vi "Test Load Virtual NEO480 cRIO XNET.vi"(11 "Test Case In":refnum<class "Test Instrument Manager.lvclass">) -> (0 "error out":errorcluster, 3 "Test Case Out":refnum<class "Test Instrument Manager.lvclass">)   [LabVIEW 2024, in "Test Instrument Manager.lvclass"]
uses:
  Test Instrument Manager.lvclass
  Test Instrument Manager.lvclass/Test Instrument Manager.ctl
  <vilib>/Astemes/LUnit/Test Case.lvclass
  Source/Instrument Manager/Instrument Manager.lvclass
  Source/Interfaces/IRead Temperature/IRead Temperature.lvclass
  Source/Interfaces/IVirtual Instrument/IVirtual Instrument.lvclass
  Source/Interfaces/IReadPressure/IRead Pressure.lvclass
  Source/Interfaces/IRead Dew Point/IRead Dew Point.lvclass
  Source/Interfaces/IRead Humidity/IRead Humidity.lvclass
  Source/Interfaces/IRead H2O Concentration/IRead H2O Concentration.lvclass
  Source/Interfaces/IRunnable/IRunnable.lvclass
panel:
  out "Time Stamp c":timestamp format="%<%x %.3X>T"
  out "H2O Concentration":dbl format="%d Vol.-%"
  out "Absolute Humidity":dbl format="%.1f g/m³"
  out "Time Stamp h":timestamp format="%<%x %.3X>T"
  out "iteration":i32
  out "Dew Point":dbl format="%.2f °C"
  out "Time Stamp d":timestamp format="%<%x %.3X>T"
  out "Time Stamp p":timestamp format="%<%x %.3X>T"
  out "Pressure":dbl format="%d mbar a"
  out "Temperature":dbl format="%.2f °C"
  out "Time Stamp t":timestamp format="%<%x %.3X>T"
  in  "stop":bool
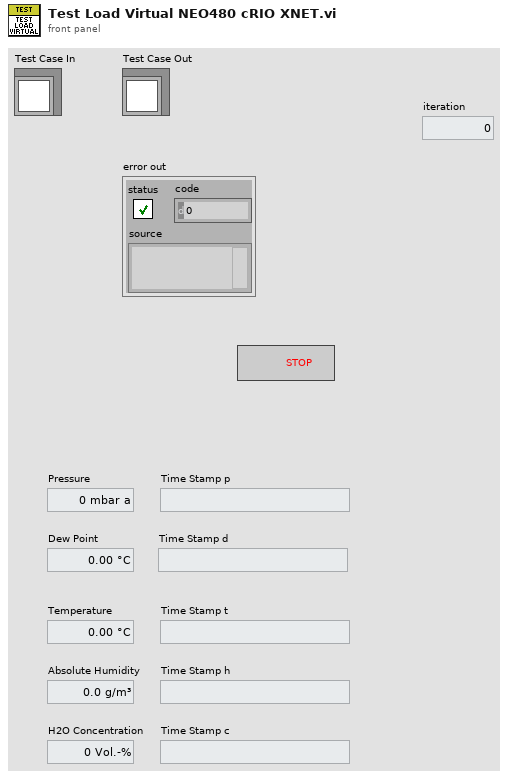
[diagram p1: front panel]
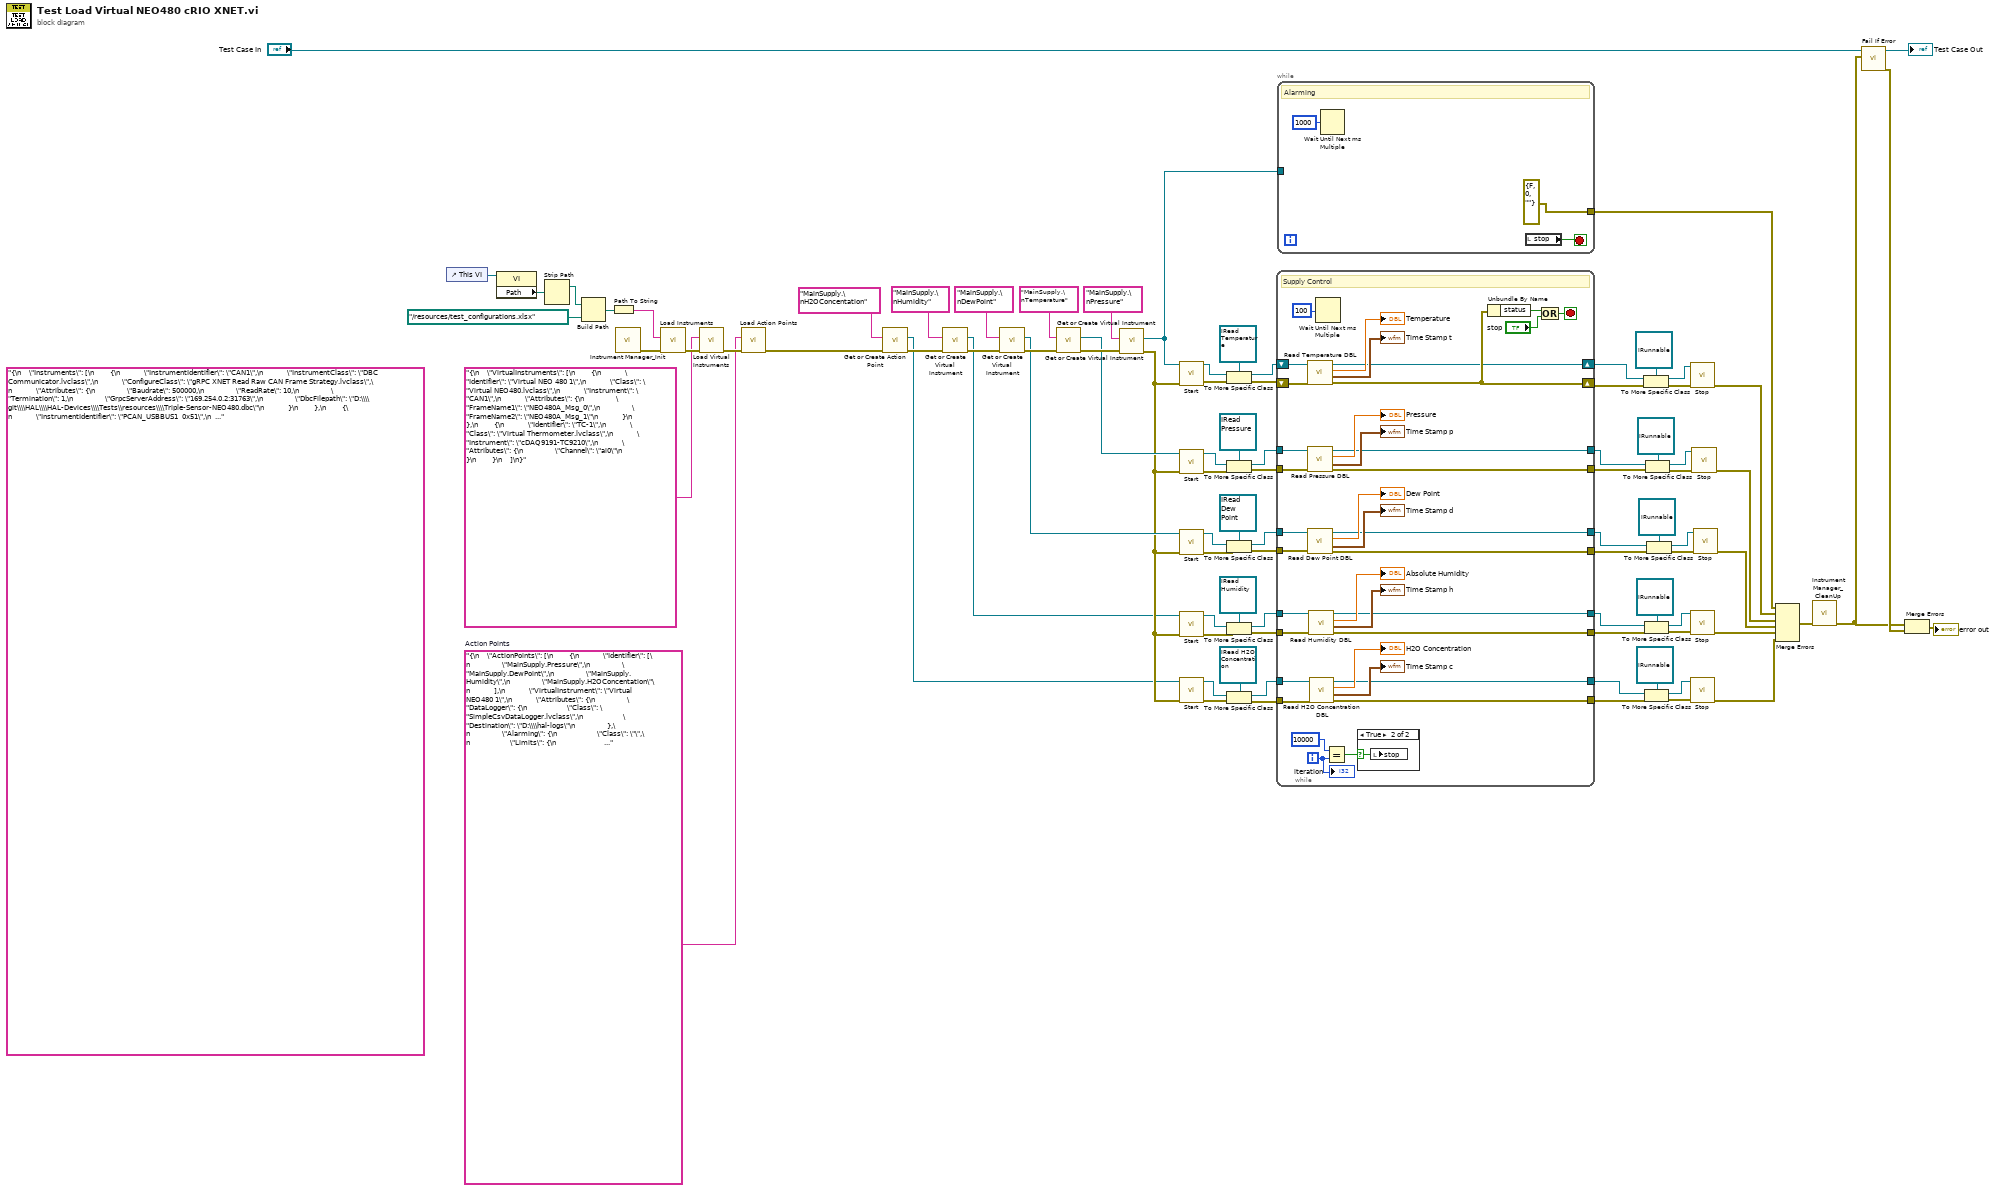
[diagram p0: block diagram]
diagram:
  w1 = "{\n    \"ActionPoints\": [\n        {\n            \"Identifier\": [\n                \"MainSupply.Pressure\",\n                \"MainSupply.DewPoint\",\n                \"MainSupply.Humidity\",\n                \"MainSupply.H2OConcentation\"\n            ],\n            \"VirtualInstrument\": \"Virtual NEO480 1\",\n            \"Attributes\": {\n                \"DataLogger\": {\n                    \"Class\": \"SimpleCsvDataLogger.lvclass\",\n                    \"Destination\": \"D:\\\\hal-logs\"\n                },\n                \"Alarming\": {\n                    \"Class\": \"\",\n                    \"Limits\": {\n                        \"Upper\": 999,\n                        \"Lower\": 0\n                    }\n                }\n            }\n        },\n        {\n            \"Identifier\": [\n                \"MainSupply.Temperature\"\n            ],\n            \"VirtualInstrument\": \"Virtual NEO480 1\",\n            \"Attributes\": {\n                \"DataLogger\": {\n                    \"Class\": \"SimpleCsvDataLogger.lvclass\",\n                    \"Destination\": \"D:\\\\hal-logs\"\n                },\n                \"Alarming\": {\n                    \"Class\": \"\",\n                    \"Limits\": {\n                        \"Upper\": 32,\n                        \"Lower\": 0\n                    }\n                }\n            }\n        }\n    ]\n}"  # Action Points
  (unwired) "{\n    \"Instruments\": [\n        {\n            \"InstrumentIdentifier\": \"CAN1\",\n            \"InstrumentClass\": \"DBC Communicator.lvclass\",\n            \"ConfigureClass\": \"gRPC XNET Read Raw CAN Frame Strategy.lvclass\",\n            \"Attributes\": {\n                \"Baudrate\": 500000,\n                \"ReadRate\": 10,\n                \"Termination\": 1,\n                \"GrpcServerAddress\": \"169.254.0.2:31763\",\n                \"DbcFilepath\": \"D:\\\\git\\\\HAL\\\\HAL-Devices\\\\Tests\\resources\\\\Triple-Sensor-NEO480.dbc\"\n            }\n        },\n        {\n            \"InstrumentIdentifier\": \"PCAN_USBBUS1  0x51\",\n            \"InstrumentClass\": \"DBC Communicator.lvclass\",\n            \"ConfigureClass\": \"PCAN Read Raw CAN Frame Strategy.lvclass\",\n            \"Attributes\": {\n                \"Baudrate\": 500000,\n                \"ReadRate\": 10,\n                \"DbcFilepath\": \"D:\\\\git\\\\HAL\\\\HAL-Devices\\\\Tests\\resources\\\\Triple-Sensor-NEO480.dbc\"\n            }\n        },\n        {\n            \"InstrumentIdentifier\": \"cDAQ9191-TC9210\",\n            \"InstrumentClass\": \"Thermometer Multichannel.lvclass\",\n            \"ConfigureClass\": \"DAQmx Thermocouple Continuous Read Strategy.lvclass\",\n            \"Attributes\": {\n                \"ReadRate\": 10,\n                \"Channels\": [\n                    {\n                        \"Name\": \"ai0\",\n                        \"Enabled\": true,\n                        \"Minimum Value\": 0,\n                        \"Maximum Value\": 100,\n                        \"Thermocouple Type\": \"J\",\n                        \"Units\": \"Deg C\",\n                        \"CJC Channel\": \"\",\n                        \"CJC Source\": \"Constant Value\",\n                        \"CJC Value\": 25\n                    }\n                ],\n                \"Timing\": {\n                    \"Type\": \"Sample Clock\",\n                    \"Samples per Channel\": 1000,\n                    \"Sample Mode\": \"Continuous Samples\",\n                    \"Sample Rate\": 10,\n                    \"Sample Clock Source\": \"OnboardClock\",\n                    \"Active Edge\": \"Rising\"\n                },\n                \"Trigger\": {\n                    \"Trigger Type\": \"No Trigger\"\n                }\n            }\n        }\n    ]\n}" ("Source")
  n1 = control-ref of="This VI"() -> (w38:refnum<vi>)
  n2 = property class="VI"(reference=w38) -> ("Path"=w37:path)  [unwired: 1 in, 2 out]
  n3 = Strip Path(path=w37) -> (stripped path=w36:path)  [unwired: 1 out]
  n4 = Build Path(base path=w36, name or relative path=path "../resources/test_configurations.xlsx") -> (appended path=w34:path)
  n5 = Path To String(path=w34) -> (string=w33:string)
  n6 = call "Instrument Manager_Init.vi"() -> ("Error Out"=w84:errorcluster)  [unwired: 10 in, 1 out]
  n7 = call "Load Instruments.vi"("Error In"=w84, "Source"=w33) -> ("Error Out"=w81:errorcluster)  [unwired: 9 in]
  n8 = call "Load Virtual Instruments.vi"("Error In"=w81, "Source"="{\n    \"VirtualInstruments\": [\n        {\n            \"Identifier\": \"Virtual NEO 480 1\",\n            \"Class\": \"Virtual NEO480.lvclass\",\n            \"Instrument\": \"CAN1\",\n            \"Attributes\": {\n                \"FrameName1\": \"NEO480A_Msg_0\",\n                \"FrameName2\": \"NEO480A_Msg_1\"\n            }\n        },\n        {\n            \"Identifier\": \"TC-1\",\n            \"Class\": \"Virtual Thermometer.lvclass\",\n            \"Instrument\": \"cDAQ9191-TC9210\",\n            \"Attributes\": {\n                \"Channel\": \"ai0\"\n            }\n        }\n    ]\n}") -> ("Error Out"=w53:errorcluster)  [unwired: 9 in]
  n9 = call "Load Action Points.vi"("Error In"=w53, "Source"=w1) -> ("Error Out"=w2:errorcluster)  [unwired: 9 in]
  n10 = call "Get or Create Action Point.vi"("Error In"=w2, "Action Point Identifier"="MainSupply.\nH2OConcentation" ("Virtual Instrument Identifier")) -> ("Error Out"=w6:errorcluster, "IAction Point"=w3:refnum<class "IVirtual Instrument.lvclass">)  [unwired: 8 in]
  n11 = call "Get or Create Virtual Instrument.vi"("Error In"=w6, "Virtual Instrument Identifier"="MainSupply.\nHumidity") -> ("Error Out"=w16:errorcluster, "IVritual Instrument"=w4:refnum<class "IVirtual Instrument.lvclass">)  [unwired: 8 in]
  n12 = call "Get or Create Virtual Instrument.vi"("Error In"=w16, "Virtual Instrument Identifier"="MainSupply.\nDewPoint" ("Instrument Identifier")) -> ("Error Out"=w52:errorcluster, "IVritual Instrument"=w48:refnum<class "IVirtual Instrument.lvclass">)  [unwired: 8 in]
  n13 = call "Get or Create Virtual Instrument.vi"("Error In"=w52, "Virtual Instrument Identifier"="MainSupply.\nTemperature") -> ("Error Out"=w79:errorcluster, "IVritual Instrument"=w54:refnum<class "IVirtual Instrument.lvclass">)  [unwired: 8 in]
  n14 = call "Get or Create Virtual Instrument.vi"("Error In"=w79, "Virtual Instrument Identifier"="MainSupply.\nPressure" ("Instrument Identifier")) -> ("Error Out"=w18:errorcluster, "IVritual Instrument"=w39:refnum<class "IVirtual Instrument.lvclass">)  [unwired: 8 in]
  n15 = call-dynamic "Start.vi"("error in"=w18, "IRunnable in"=w39) -> ("error out"=w72:errorcluster, "IRunnable out"=w73:refnum<class "IVirtual Instrument.lvclass">)  [unwired: 8 in]
  n16 = call-dynamic "Start.vi"("error in"=w18, "IRunnable in"=w54) -> ("error out"=w69:errorcluster, "IRunnable out"=w68:refnum<class "IVirtual Instrument.lvclass">)  [unwired: 8 in]
  n17 = call-dynamic "Start.vi"("error in"=w18, "IRunnable in"=w48) -> ("error out"=w59:errorcluster, "IRunnable out"=w60:refnum<class "IVirtual Instrument.lvclass">)  [unwired: 8 in]
  n18 = call-dynamic "Start.vi"("error in"=w18, "IRunnable in"=w4) -> ("error out"=w31:errorcluster, "IRunnable out"=w30:refnum<class "IVirtual Instrument.lvclass">)  [unwired: 8 in]
  n19 = call-dynamic "Start.vi"("error in"=w18, "IRunnable in"=w3) -> ("error out"=w19:errorcluster, "IRunnable out"=w17:refnum<class "IVirtual Instrument.lvclass">)  [unwired: 8 in]
  n20 = To More Specific Class(target class=refnum<class "IRead Temperature.lvclass"> refnum ("IRead Temperature.lvclass"), reference=w73, error in=w72) -> (specific class reference=w70:refnum<class "IRead Temperature.lvclass">, error out=w71:errorcluster)
  n21 = To More Specific Class(target class=refnum<class "IRead Pressure.lvclass"> refnum ("IRead Pressure.lvclass"), reference=w68, error in=w69) -> (specific class reference=w56:refnum<class "IRead Pressure.lvclass">, error out=w55:errorcluster)
  n22 = To More Specific Class(target class=refnum<class "IRead Dew Point.lvclass"> refnum ("IRead Dew Point.lvclass"), reference=w60, error in=w59) -> (specific class reference=w57:refnum<class "IRead Dew Point.lvclass">, error out=w58:errorcluster)
  n23 = To More Specific Class(target class=refnum<class "IRead Humidity.lvclass"> refnum ("IRead Humidity.lvclass"), reference=w30, error in=w31) -> (specific class reference=w27:refnum<class "IRead Humidity.lvclass">, error out=w28:errorcluster)
  n24 = To More Specific Class(target class=refnum<class "IRead H2O Concentration.lvclass"> refnum ("IRead H2O Concentration.lvclass"), reference=w17, error in=w19) -> (specific class reference=w15:refnum<class "IRead H2O Concentration.lvclass">, error out=w20:errorcluster)
  n25 = while {
    shift-right: [w118] -> w77
    shift-left: w70 -> [w116]
    shift-right: [w119] -> w86
    shift-left: w71 -> [w117]
    tunnel: w58 -> [w110]
    tunnel: w57 -> [w109]
    tunnel: w56 -> [w108]
    tunnel: w55 -> [w107]
    tunnel: [w106] -> w41
    tunnel: [w105] -> w42
    tunnel: [w104] -> w43
    tunnel: [w103] -> w44
    tunnel: w28 -> [w101]
    tunnel: w27 -> [w100]
    tunnel: [w99] -> w26
    tunnel: [w96] -> w25
    tunnel: w20 -> [w95]
    tunnel: [w92] -> w10
    tunnel: w15 -> [w91]
    tunnel: [w90] -> w9
    i -> [w102]
    stop <- w123 stop-if-true
    # "Supply Control"
    n26 = call-dynamic "Read Temperature DBL.vi"("error in"=w117, "IRead Temperature in"=w116) -> ("error out"=w119:errorcluster, "Time Stamp"=→"Time Stamp t":timestamp, "Temperature"=→"Temperature":dbl, "IRead Temperature out"=w118:refnum<class "IRead Temperature.lvclass">)  [unwired: 6 in]
    n27 = call-dynamic "Read Pressure DBL.vi"("error in"=w107, "IRead Pressure in"=w108) -> ("error out"=w106:errorcluster, "Time Stamp"=→"Time Stamp p":timestamp, "Pressure"=→"Pressure":dbl, "IRead Pressure out"=w105:refnum<class "IRead Pressure.lvclass">)  [unwired: 6 in]
    n28 = call-dynamic "Read Dew Point DBL.vi"("error in"=w110, "IRead Dew Point in"=w109) -> ("error out"=w103:errorcluster, "Time Stamp"=→"Time Stamp d":timestamp, "Dew Point"=→"Dew Point":dbl, "IRead Dew Point out"=w104:refnum<class "IRead Dew Point.lvclass">)  [unwired: 6 in]
    n29 = call-dynamic "Read Humidity DBL.vi"("error in"=w101, "IRead Absolute Humidity in"=w100) -> ("error out"=w99:errorcluster, "Time Stamp"=→"Time Stamp h":timestamp, "Humidity"=→"Absolute Humidity":dbl, "IRead Absolute Humidity out"=w96:refnum<class "IRead Humidity.lvclass">)  [unwired: 6 in]
    n30 = call-dynamic "Read H2O Concentration DBL.vi"("error in"=w95, "IRead Water Concentration in"=w91) -> ("error out"=w92:errorcluster, "Time Stamp"=→"Time Stamp c":timestamp, "H2O Concentration"=→"H2O Concentration":dbl, "IRead Water Concentration out"=w90:refnum<class "IRead H2O Concentration.lvclass">)  [unwired: 6 in]
    n31 = Wait Until Next ms Multiple(millisecond multiple=u32 100) -> ()  [unwired: 1 out]
    n32 = Equal?(x=10000, y=w102) -> (x = y?=w115:bool)
    n33 = case shown="True" w115 {
      selector: w115 -> [_ w127]
      frame False {
      }
      frame True {
        n34 = local write "stop"(w127) -> ()
      }
    }
    n35 = Unbundle By Name(w119) -> ("status"=w120:bool)
    n36 = Or(x=w120, y="stop") -> (x .or. y?=w123:bool)
    "iteration" <- w102
  }
  n37 = while {
    tunnel: w39 -> [_]
    tunnel: [errorcluster {"status"=FALSE, "code"=0, "source"=""} ("error constant")] -> w32
    stop <- w129 stop-if-true
    # "Alarming"
    n38 = Wait Until Next ms Multiple(millisecond multiple=u32 1000) -> ()  [unwired: 1 out]
    n39 = local read "stop"() -> (w129:bool)
  }
  n40 = To More Specific Class(target class=refnum<class "IRunnable.lvclass"> refnum ("IRunnable.lvclass"), reference=w77, error in=w86) -> (specific class reference=w75:refnum<class "IRunnable.lvclass">, error out=w78:errorcluster)
  n41 = To More Specific Class(target class=refnum<class "IRunnable.lvclass"> refnum ("IRunnable.lvclass"), reference=w25, error in=w26) -> (specific class reference=w22:refnum<class "IRunnable.lvclass">, error out=w24:errorcluster)
  n42 = To More Specific Class(target class=refnum<class "IRunnable.lvclass"> refnum ("IRunnable.lvclass"), reference=w9, error in=w10) -> (specific class reference=w12:refnum<class "IRunnable.lvclass">, error out=w11:errorcluster)
  n43 = To More Specific Class(target class=refnum<class "IRunnable.lvclass"> refnum ("IRunnable.lvclass"), reference=w42, error in=w41) -> (specific class reference=w66:refnum<class "IRunnable.lvclass">, error out=w64:errorcluster)
  n44 = To More Specific Class(target class=refnum<class "IRunnable.lvclass"> refnum ("IRunnable.lvclass"), reference=w43, error in=w44) -> (specific class reference=w45:refnum<class "IRunnable.lvclass">, error out=w47:errorcluster)
  n45 = call-dynamic "Stop.vi"("error in"=w78, "IRunnable in"=w75) -> ("error out"=w83:errorcluster)  [unwired: 8 in, 1 out]
  n46 = call-dynamic "Stop.vi"("error in"=w24, "IRunnable in"=w22) -> ("error out"=w23:errorcluster)  [unwired: 8 in, 1 out]
  n47 = call-dynamic "Stop.vi"("error in"=w11, "IRunnable in"=w12) -> ("error out"=w8:errorcluster)  [unwired: 8 in, 1 out]
  n48 = call-dynamic "Stop.vi"("error in"=w64, "IRunnable in"=w66) -> ("error out"=w62:errorcluster)  [unwired: 8 in, 1 out]
  n49 = call-dynamic "Stop.vi"("error in"=w47, "IRunnable in"=w45) -> ("error out"=w40:errorcluster)  [unwired: 8 in, 1 out]
  n50 = Merge Errors(w32, w83, w62, w40, w23, w8) -> (w63:errorcluster)
  n51 = call "Instrument Manager_CleanUp.vi"("Error In"=w63) -> ("Error Out"=w82:errorcluster)  [unwired: 10 in]
  n52 = call <vilib>:"Fail If Error.vi"("Assert error"=w82, "LUnit Test Case In"="Test Case In") -> ("error out"=w87:errorcluster, "LUnit Test Case Out"=→"Test Case Out":refnum<class "Test Instrument Manager.lvclass">)  [unwired: 8 in]
  n53 = Merge Errors(w82, w87) -> (→"error out":errorcluster)
